vi "Update Preview.vi"(8 "error in (no error)":errorcluster, 11 "Recipe Editor in":refnum<class "Recipe Editor.lvclass">) -> (0 "error out":errorcluster, 3 "Recipe Editor out":refnum<class "Recipe Editor.lvclass">)   [LabVIEW 2018, in "Temp Recipe.lvlib" / "Recipe Editor.lvclass"]
uses:
  Recipe Editor.lvclass
  Update Event Data.ctl
  Recipe Editor.lvclass/Recipe Editor.ctl
  Temp Recipe.lvlib
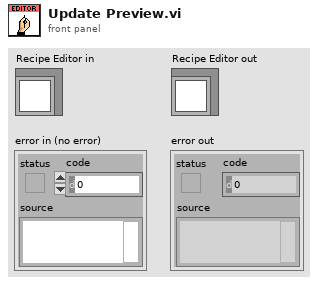
[diagram p1: front panel]
types:
  T1 = typedef "Temp Recipe.lvlib/Update Event Data.ctl" = bool
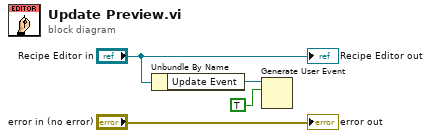
[diagram p0: block diagram]
diagram:
  n1 = Unbundle By Name("Recipe Editor in") -> ("Update Event"=w2:refnum<user-event>)
  n2 = Generate User Event(user event=w2, event data cluster=T1 TRUE ("event data")) -> ()  [unwired: 2 in, 2 out]
  "error out" <- "error in (no error)"
  "Recipe Editor out" <- "Recipe Editor in"
